vi "Transfer Viewable Resources.vi"(10 "Recipient Viewable In":refnum<class "IViewable.lvclass">, 11 "Running Viewable":refnum<class "IViewable.lvclass">) -> (2 "Recipient Viewable Out":refnum<class "IViewable.lvclass">)   [LabVIEW 2017, in "IViewable.lvlib" / "IViewable.lvclass"]
uses:
  IViewable.lvclass
  C:/Git/mva-framework/Source/Framework/IObserver/IObserver/IObserver.lvclass
  IViewable.lvclass/IViewable.ctl
  IObserver/IObserver/IObserver.lvclass/IObserver.ctl
  IObserver/IObserver/IObserver.lvclass
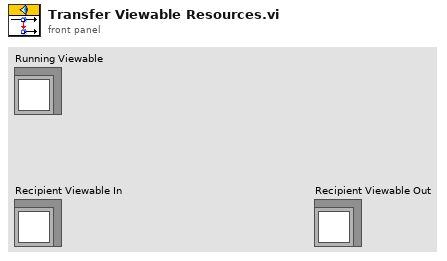
[diagram p1: front panel]
types:
  T1 = typedef "IViewable.lvlib/ApplicationStyleReference.lvclass/Application Style Reference.ctl" = refnum<data-value>
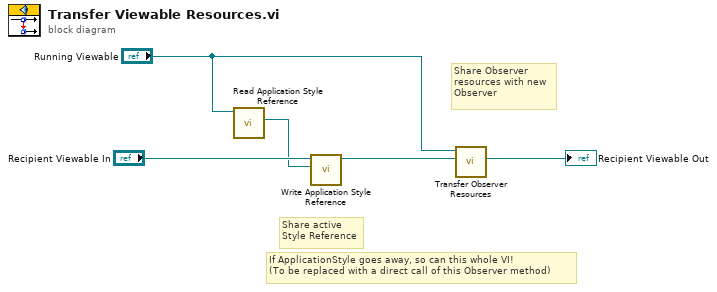
[diagram p0: block diagram]
diagram:
  # "If ApplicationStyle goes away, so can this whole VI!\n(To be replaced with a direct call of this Observer method)"
  # "Share Observer\nresources with new\nObserver"
  # "Share active\nStyle Reference"
  n1 = call "Read Application Style Reference.vi"("IViewable in"="Running Viewable") -> ("Application Style Reference"=w4:T1)  [unwired: 10 in]
  n2 = call "Write Application Style Reference.vi"("Application Style Reference"=w4, "IViewable in"="Recipient Viewable In") -> ("IViewable out"=w2:refnum<class "IViewable.lvclass">)  [unwired: 9 in]
  n3 = call "Transfer Observer Resources.vi"("Recipient Observer In"=w2, "Running Observer"="Running Viewable") -> ("Recipient Observer Out"=→"Recipient Viewable Out":refnum<class "IViewable.lvclass">)  [unwired: 9 in]
